vi "init.vi"(0 "VISA Refnum in":refnum<visa-resource-name>) -> (17 "array of ranges":cluster{"low":dbl, "high":dbl}[](array[cluster]), 20 "VISA out":refnum<visa-resource-name>, 21 "HTTP client handle out":T1, 24 "Internet OK":bool, 26 "HTTP client error out":errorcluster, 27 "VISA error out":errorcluster)   [LabVIEW 2016]
uses:
  <vilib>/httpClient/ClientHandle.ctl
  <vilib>/Instr/_visa.llb/VISA Configure Serial Port (Instr).vi
  <vilib>/httpClient/LabVIEWHTTPClient.lvlib
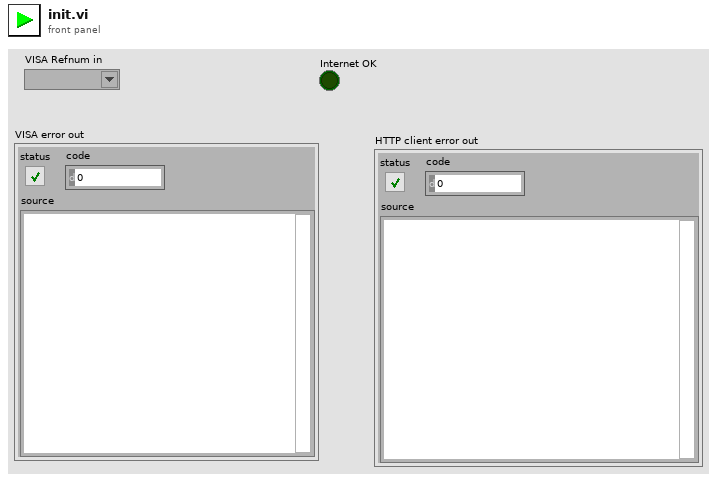
[diagram p1: front panel]
types:
  T1 = typedef "LabVIEWHTTPClient.lvlib/ClientHandle.ctl" = refnum<k1>
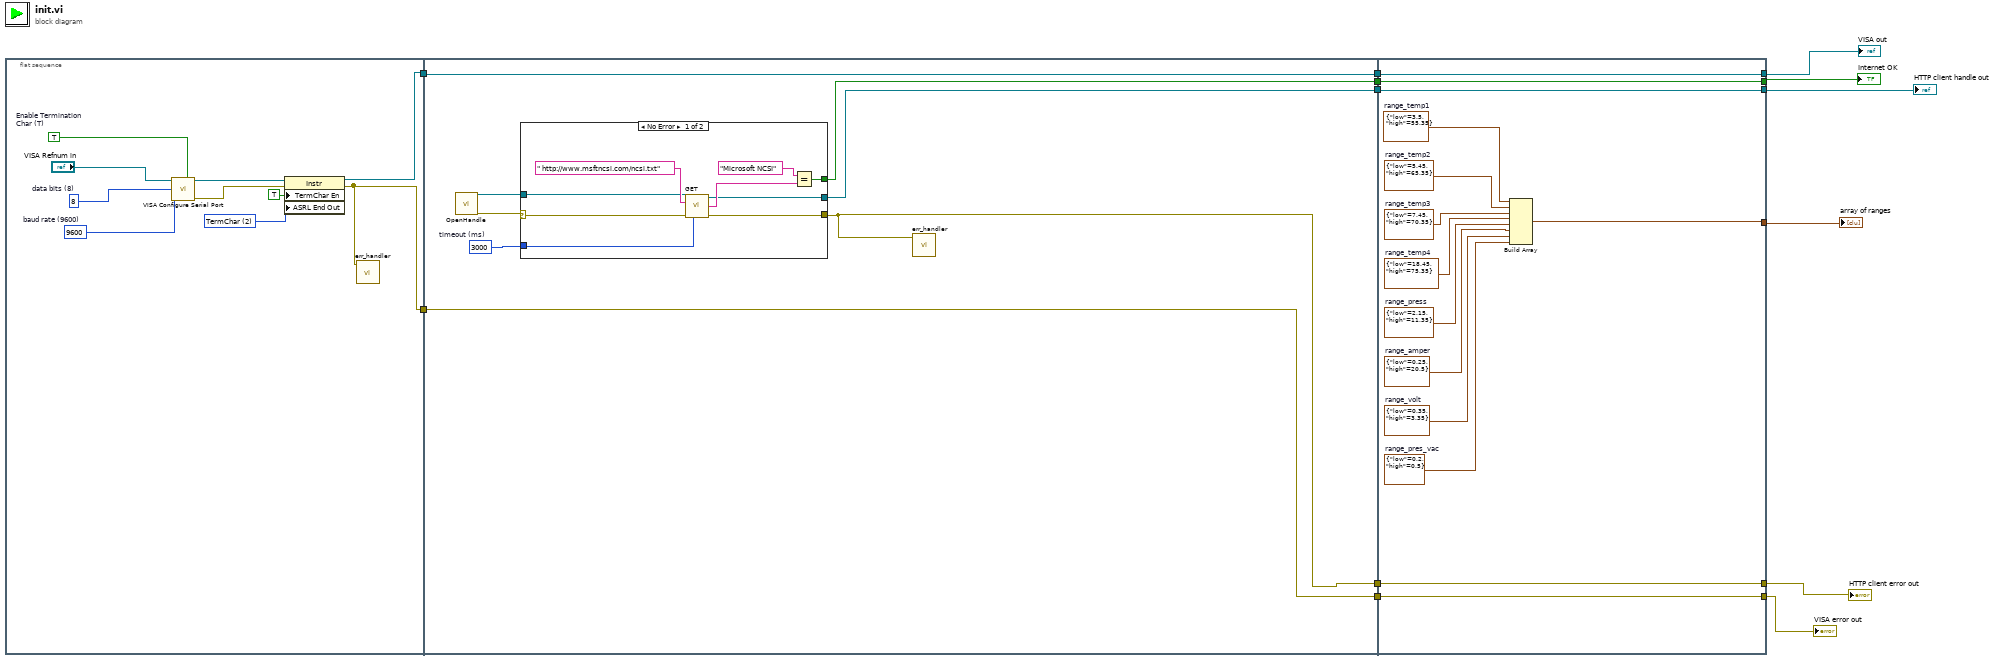
[diagram p0: block diagram]
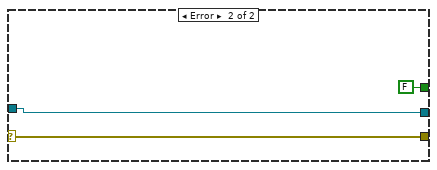
[diagram p2: hidden frame]
diagram:
  n1 = flat-sequence {
    tunnel: [w15] -> w13
    tunnel: [w14] -> w1
    tunnel: [w31] -> w11
    tunnel: [w30] -> w10
    tunnel: [w29] -> w9
    tunnel: [w28] -> w8
    tunnel: [w27] -> w7
    tunnel: w1 -> [w27]
    tunnel: w13 -> [w31]
    tunnel: [w55] -> w4
    tunnel: [w56] -> w12
    tunnel: [w57] -> w3
    tunnel: w11 -> [w57]
    tunnel: w10 -> [w56]
    tunnel: w9 -> [w55]
    tunnel: w8 -> [w45]
    tunnel: w7 -> [w46]
    tunnel: [w46] -> w5
    tunnel: [w45] -> w6
    tunnel: [w44] -> w2
    frame #0 {
      w17 = u16 2 items=["None", "Last Bit", "TermChar", "Break"] ("Serial Settings:End Mode for Writes")
      w20 = u16 8  # data bits (8)
      w21 = TRUE  # Enable Termination Char (T)
      w22 = u32 9600  # baud rate (9600)
      n2 = call-poly "VISA Configure Serial Port"("VISA resource name"="VISA Refnum in", "Enable Termination\nChar (T)"=w21, "baud rate (9600)"=w22, "data bits (8)"=w20) -> ("VISA resource name out"=w19:refnum<visa-resource-name>, "error out"=w16:errorcluster)  [unwired: 10 in]
      n3 = property class="Instr"(reference=w19, error in=w16, "TermChar En"=TRUE ("Message Based Settings:Termination Character Enable"), "ASRL End Out"=w17) -> (reference out=w15:refnum<visa-resource-name>, error out=w14:errorcluster)
      n4 = call "err_handler.vi"("error in (no error)"=w14) -> ()  [unwired: 11 in]
    }
    frame #1 {
      w26 = 3000  # timeout (ms)
      n5 = call <vilib>:"OpenHandle.vi"() -> ("client handle out"=w24:T1, "error out"=w25:errorcluster)  [unwired: 14 in]
      n6 = case shown="No Error" w25 {
        selector: w25 -> [w35 w42]
        tunnel: [w37 FALSE] -> w30
        tunnel: [w36 w42] -> w28
        tunnel: w26 -> [w34 _]
        tunnel: w24 -> [w33 w41]
        tunnel: [w32 w41] -> w29
        frame No Error {
          n7 = call <vilib>:"GET.vi"("client handle"=w33, "url"=" http://www.msftncsi.com/ncsi.txt" ("address"), "error in (no error)"=w35, "timeout (10000)"=w34) -> ("client handle out"=w32:T1, "body"=w38:string, "error out"=w36:errorcluster)  [unwired: 8 in, 1 out]
          n8 = Equal?(x="Microsoft NCSI", y=w38) -> (x = y?=w37:bool)
        }
        frame Error {
        }
      }
      n9 = call "err_handler.vi"("error in (no error)"=w28) -> ()  [unwired: 11 in]
    }
    frame #2 {
      w47 = cluster{"low":dbl, "high":dbl} {"low"=0.2, "high"=0.5}  # range_pres_vac
      w48 = cluster{"low":dbl, "high":dbl} {"low"=0.35, "high"=3.35}  # range_volt
      w49 = cluster{"low":dbl, "high":dbl} {"low"=0.25, "high"=20.5}  # range_amper
      w50 = cluster{"low":dbl, "high":dbl} {"low"=2.15, "high"=11.35}  # range_press
      w51 = cluster{"low":dbl, "high":dbl} {"low"=18.45, "high"=75.35}  # range_temp4
      w52 = cluster{"low":dbl, "high":dbl} {"low"=7.45, "high"=70.35}  # range_temp3
      w53 = cluster{"low":dbl, "high":dbl} {"low"=5.45, "high"=65.35}  # range_temp2
      w54 = cluster{"low":dbl, "high":dbl} {"low"=3.5, "high"=55.35}  # range_temp1
      n10 = Build Array(w54, w53, w52, w51, w50, w49, w48, w47) -> (w44:cluster{"low":dbl, "high":dbl}[])
    }
  }
  "VISA out" <- w3
  "VISA error out" <- w5
  "Internet OK" <- w12
  "HTTP client handle out" <- w4
  "HTTP client error out" <- w6
  "array of ranges" <- w2
